vi "Read_Dataset(asIn3D_Out1D).vi"(0 "Image Folder Path(Train)":path, 1 "Norm. Shift":sgl=65535.0, 3 "Norm. Scale":sgl=65535.0, 5 "Label File Path(Train)":path, 7 "Image Folder Path(Test)":path, 9 "Label File Path(Test)":path, 11 "error in (no error)":errorcluster, 12 "Img Heigth":i32=-1, 14 "Img Width":i32=-1) -> (4 "Datasets":T1, 15 "error out":errorcluster)   [LabVIEW 2020]
doc: "Referecens to the dataset (Trainining, Validation and Testing)"
uses:
  <vilib>/Ngene/DeepLTK/Toolkit/NN_Data/API/DataSet_Types/NN_DataSets_All(In3D_Out1D).ctl
  <vilib>/Ngene/DeepLTK/Toolkit/NN_Data/API/DataSet_Types/NN_DataSet(In3D_Out1D).ctl
  <vilib>/Ngene/DeepLTK/Toolkit/NN_Data/API/DataRef_Types/NN_Data_ref(4D_SGL).ctl
  <vilib>/Ngene/DeepLTK/Toolkit/NN_Data/API/DataRef_Types/NN_Data_ref(2D_SGL).ctl
  <vilib>/Ngene/DeepLTK/Toolkit/NN_Data/API/DataRef_Types/NN_Data_ref(1D_I32).ctl
  <vilib>/Ngene/DeepLTK/Toolkit/NN_Data/Controls/NN_Dims(C,H,W).ctl
  <vilib>/Ngene/DeepLTK/Toolkit/Deep_Learning_Toolkit_by_Ngene.lvlib
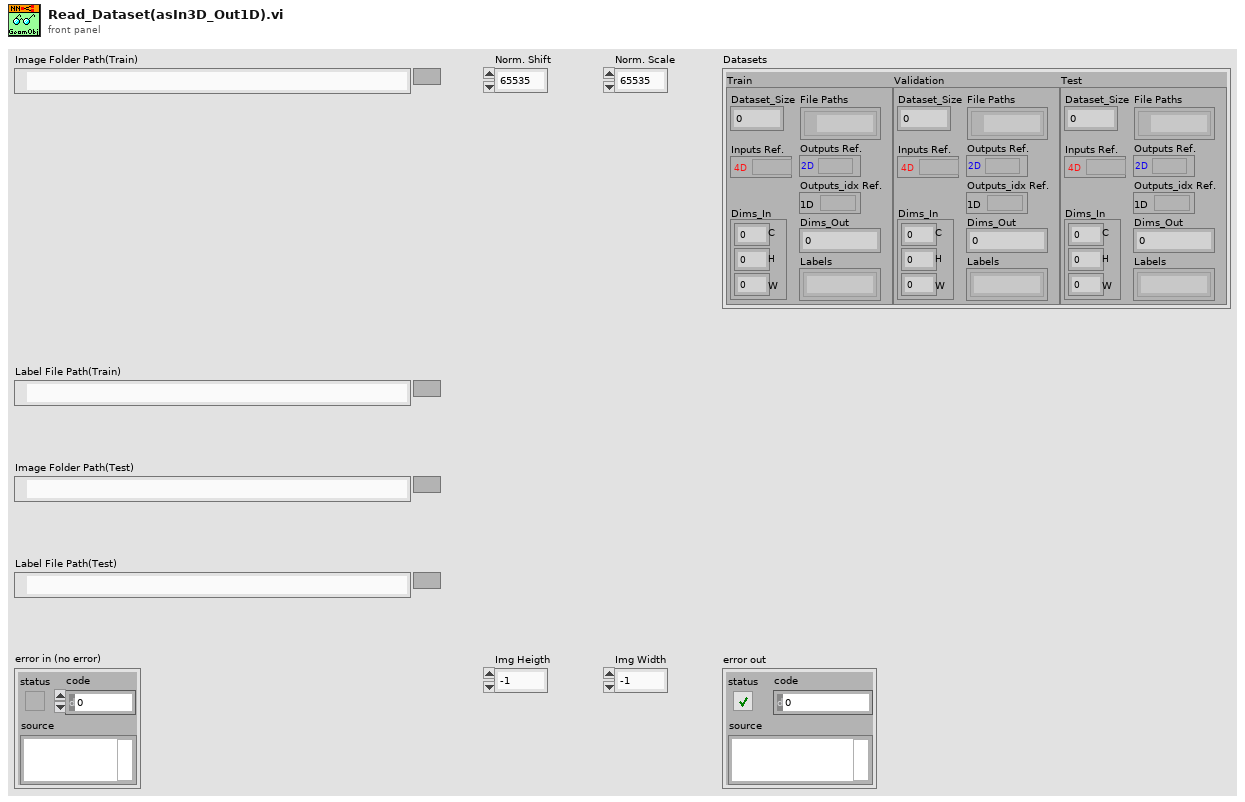
[diagram p1: front panel]
types:
  T1 = typedef "Deep_Learning_Toolkit_by_Ngene.lvlib/NN_DataSets_All(In3D_Out1D).ctl" = cluster{"Train":T2, "Validation":T2, "Test":T2}
  T2 = typedef "Deep_Learning_Toolkit_by_Ngene.lvlib/NN_DataSet(In3D_Out1D).ctl" = cluster{"Inputs Ref.":T3, "Outputs Ref.":T4, "Dataset_Size":i32, "Outputs_idx Ref.":T5, "Dims_In":T6, "Dims_Out":i32, "Labels":string[], "File Paths":path[]}
  T3 = typedef "Deep_Learning_Toolkit_by_Ngene.lvlib/NN_Data_ref(4D_SGL).ctl" = refnum<data-value>
  T4 = typedef "Deep_Learning_Toolkit_by_Ngene.lvlib/NN_Data_ref(2D_SGL).ctl" = refnum<data-value>
  T5 = typedef "Deep_Learning_Toolkit_by_Ngene.lvlib/NN_Data_ref(1D_I32).ctl" = refnum<data-value>
  T6 = typedef "Deep_Learning_Toolkit_by_Ngene.lvlib/NN_Dims(C,H,W).ctl" = cluster{"C":i32, "H":i32, "W":i32}
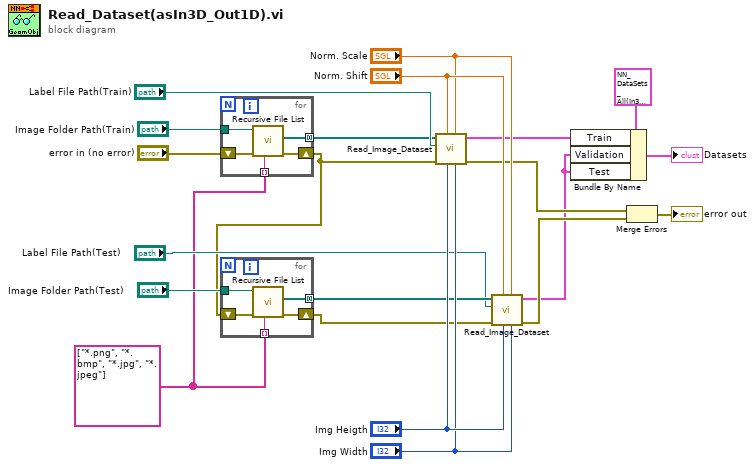
[diagram p0: block diagram]
diagram:
  w2 = string[] ["*.png", "*.bmp", "*.jpg", "*.jpeg"] ("pattern")
  n1 = for {
    tunnel: w2 -> [w26] mode=indexing
    tunnel: "Image Folder Path(Train)" -> [w24]
    tunnel: [w23] -> w10 mode=concatenating
    shift-right: [w22] -> w3
    shift-left: "error in (no error)" -> [w25]
    n2 = call <vilib>:"Recursive File List.vi"("pattern"=w26, "error in (no error)"=w25, "Folder Path"=w24) -> ("error out"=w22:errorcluster, "All Files in Dir"=w23:path[])  [unwired: 4 in, 3 out]
  }
  n3 = for {
    tunnel: w2 -> [w31] mode=indexing
    tunnel: "Image Folder Path(Test)" -> [w29]
    tunnel: [w28] -> w7 mode=concatenating
    shift-right: [w27] -> w8
    shift-left: w3 -> [w30]
    n4 = call <vilib>:"Recursive File List.vi"("pattern"=w31, "error in (no error)"=w30, "Folder Path"=w29) -> ("error out"=w27:errorcluster, "All Files in Dir"=w28:path[])  [unwired: 4 in, 3 out]
  }
  n5 = call "Read_Image_Dataset.vi"("Img Width"="Img Width", "Norm. Scale"="Norm. Scale", "Img Heigth"="Img Heigth", "Norm. Shift"="Norm. Shift", "error in (no error)"=w3, "Annotation file"="Label File Path(Train)", "Image File Paths"=w10) -> ("error out"=w4:errorcluster, "Dataset"=w12:T2)  [unwired: 3 in]
  n6 = call "Read_Image_Dataset.vi"("Img Width"="Img Width", "Norm. Scale"="Norm. Scale", "Img Heigth"="Img Heigth", "Norm. Shift"="Norm. Shift", "error in (no error)"=w8, "Annotation file"="Label File Path(Test)", "Image File Paths"=w7) -> ("error out"=w13:errorcluster, "Dataset"=w1:T2)  [unwired: 3 in]
  n7 = Bundle By Name(cluster=T1 {"Train"={"Inputs Ref."=refnum, "Outputs Ref."=refnum, "Dataset_Size"=0, "Outputs_idx Ref."=refnum, "Dims_In"={"C"=0, "H"=0, "W"=0}, "Dims_Out"=0, "Labels"=[], "File Paths"=[]}, "Validation"={"Inputs Ref."=refnum, "Outputs Ref."=refnum, "Dataset_Size"=0, "Outputs_idx Ref."=refnum, "Dims_In"={"C"=0, "H"=0, "W"=0}, "Dims_Out"=0, "Labels"=[], "File Paths"=[]}, "Test"={"Inputs Ref."=refnum, "Outputs Ref."=refnum, "Dataset_Size"=0, "Outputs_idx Ref."=refnum, "Dims_In"={"C"=0, "H"=0, "W"=0}, "Dims_Out"=0, "Labels"=[], "File Paths"=[]}} ("Dataset_Refs_All(In3D_Out1D)"), "Train"=w12, "Validation"=w1, "Test"=w1) -> (→"Datasets":T1)
  n8 = Merge Errors(w4, w13) -> (→"error out":errorcluster)
